vi "GetCurrentPosition.vi"(0 "error in":errorcluster, 5 "Telnet":refnum<k24>) -> (4 "error out":errorcluster, 6 "KclCommand":string, 8 "Succeed":bool, 10 "ErrorText":string, 15 "Position":T1)   [LabVIEW 2019, in "UnderAutomation.Fanuc.lvlib"]
uses:
  UnderAutomation.Fanuc.lvlib
  C:/Users/fg/Documents/Fanuc.vi/LabVIEW_2024/UnderAutomation.Fanuc/lib/UnderAutomation.Fanuc.dll
  LabVIEW_2024/UnderAutomation.Fanuc/lib/UnderAutomation.Fanuc.dll
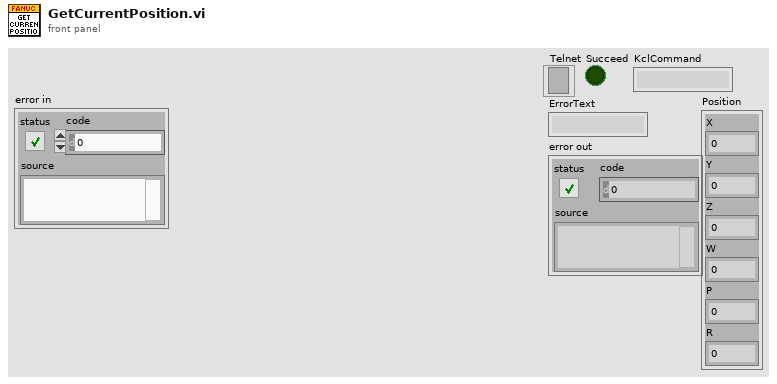
[diagram p1: front panel]
types:
  T1 = cluster{"X":dbl, "Y":dbl, "Z":dbl, "W":dbl, "P":dbl, "R":dbl}
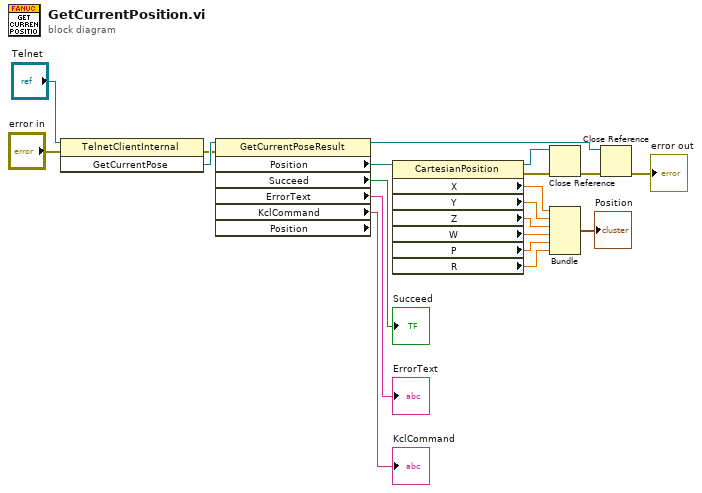
[diagram p0: block diagram]
diagram:
  n1 = invoke class="TelnetClientInternal" method="GetCurrentPose"(reference="Telnet", error in="error in") -> (error out=w16:errorcluster, "GetCurrentPose"=w19:refnum<k24>)  [unwired: 1 in, 1 out]
  n2 = property class="GetCurrentPoseResult" props=["Position", "Succeed", "ErrorText", "KclCommand", "Position"](reference=w19, error in=w16) -> (reference out=w14:refnum<k24>, "Position"=w4:refnum<k24>, "Succeed"=→"Succeed":bool, "ErrorText"=→"ErrorText":string, "KclCommand"=→"KclCommand":string)  [unwired: 2 out]
  n3 = property class="CartesianPosition"(reference=w4) -> (reference out=w5:refnum<k24>, error out=w3:errorcluster, "X"=w12:dbl, "Y"=w11:dbl, "Z"=w10:dbl, "W"=w9:dbl, "P"=w8:dbl, "R"=w7:dbl)  [unwired: 1 in]
  n4 = Close Reference(reference=w5, error in (no error)=w3) -> (error out=w2:errorcluster)
  n5 = Bundle("X"=w12, "Y"=w11, "Z"=w10, "W"=w9, "P"=w8, "R"=w7) -> (→"Position":T1)  [unwired: 1 in]
  n6 = Close Reference(reference=w14, error in (no error)=w2) -> (error out=→"error out":errorcluster)
